vi "calculateNumber.vi"(0 "Array":dbl[](array[numeric]), 1 "Drop Time (s)":dbl, 2 "abs cross section (um^2)":dbl, 3 "pixel size (um)":dbl) -> (8 "Number":dbl, 9 "Temperature (K) x":dbl format="%#_6p", 10 "Temperature (K) y":dbl format="%#_6p")   [LabVIEW 2016]
panel:
  out "alpha bar":dbl
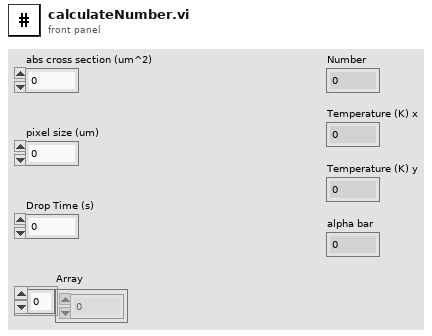
[diagram p1: front panel]
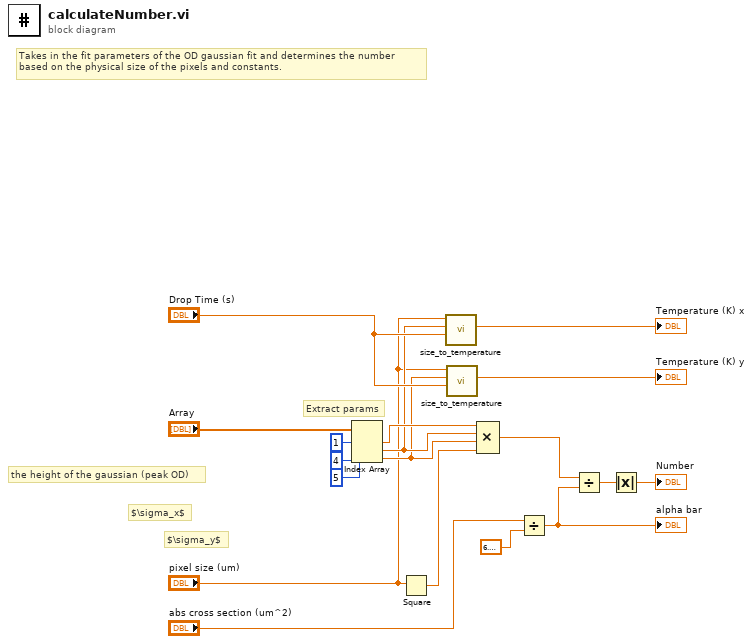
[diagram p0: block diagram]
diagram:
  # "Extract params"
  # "Takes in the fit parameters of the OD gaussian fit and determines the number\nbased on the physical size of the pixels and constants."
  # "$\\sigma_y$"
  # "$\\sigma_x$"
  # "the height of the gaussian (peak OD)"
  n1 = Index Array(array="Array", index #1=1 ("index"), index #2=4 ("index"), index #3=5 ("index")) -> (element #1=w14:dbl, element #2=w11:dbl, element #3=w10:dbl)
  n2 = Square(x="pixel size (um)") -> (x^2=w3:dbl)
  n3 = call "size_to_temperature.vi"("Drop Time"="Drop Time (s)", "sigma"=w11, "Pixel Size"="pixel size (um)") -> ("Temperature (K)"=→"Temperature (K) x":dbl)  [unwired: 8 in]
  n4 = call "size_to_temperature.vi"("Drop Time"="Drop Time (s)", "sigma"=w10, "Pixel Size"="pixel size (um)") -> ("Temperature (K)"=→"Temperature (K) y":dbl)  [unwired: 8 in]
  n5 = Compound Arithmetic op=MULTIPLY(w14, w11, w10, w3) -> (w13:dbl)
  n6 = Divide(x="abs cross section (um^2)", y=6.283185307179586) -> (x/y=w5:dbl)
  "alpha bar" <- w5
  n7 = Divide(x=w13, y=w5) -> (x/y=w2:dbl)
  n8 = Absolute Value(x=w2) -> (abs(x)=→"Number":dbl)
